vi "LB_AssertDisabledItems_Tests.vi"(11 "error in":errorcluster) -> (15 "error out":errorcluster)   [LabVIEW 2016, in "DronaTest.lvlib"]
uses:
  DronaTest.lvlib
  APIs/Stimulus/ControlValue/SetValueAuto.vi
  APIs/Assert/AssertControlValue/Controls/Listbox/AssertDisabledItems.vi
  <vilib>/addons/_JKI Toolkits/Caraya/classes/Assert/Assert Error.vi
  <vilib>/addons/_JKI Toolkits/Caraya/classes/Assert/Assert Equal Value_Variant.vi
  <vilib>/addons/_JKI Toolkits/Caraya/classes/Test/Test.lvclass
  Drona.lvlib
  <vilib>/SLL Toolkit/SLL Debug/SLL Debug.lvlib
  <vilib>/addons/_JKI Toolkits/Caraya/classes/Assert/Assert.lvclass
  APIs/Stimulus/ControlValue/ControlValue.lvlib
  APIs/Assert/AssertControlValue/Controls/Listbox/AssertListbox.lvlib
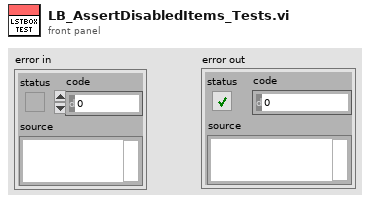
[diagram p1: front panel]
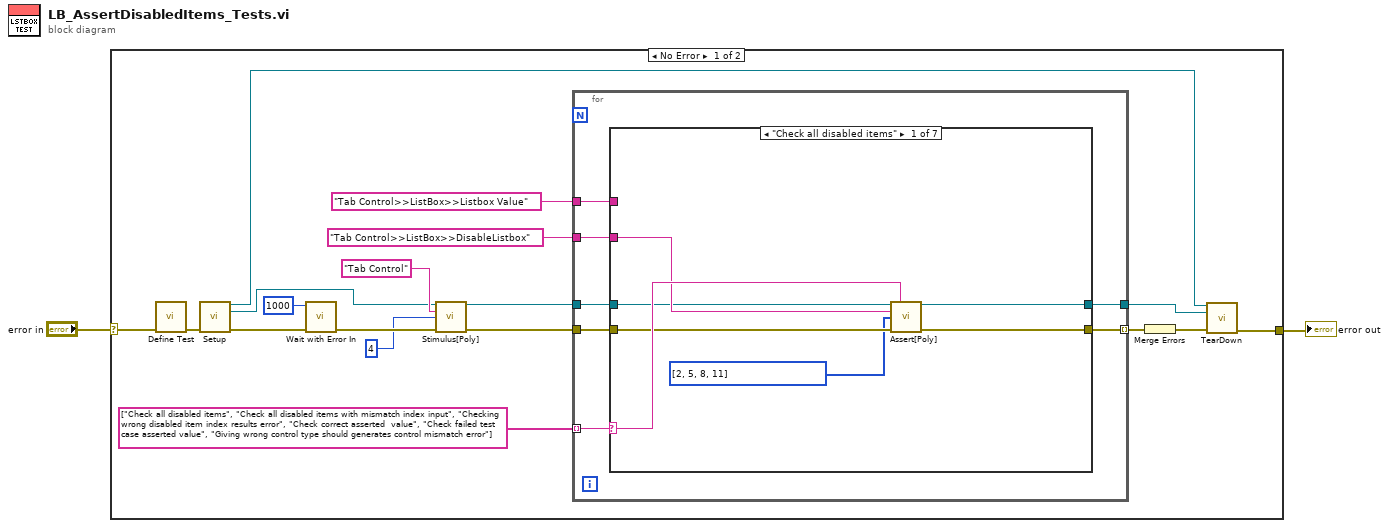
[diagram p0: block diagram]
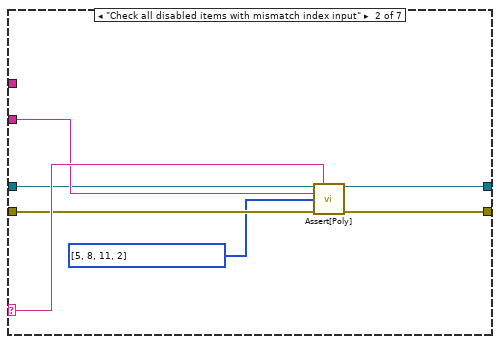
[diagram p2: hidden frame]
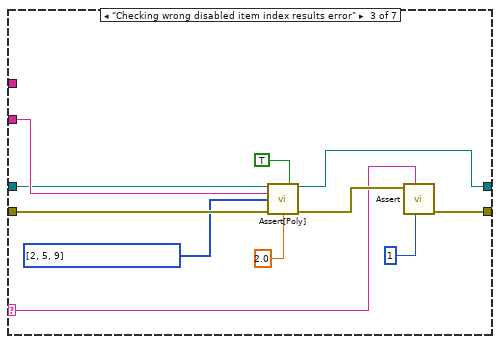
[diagram p3: hidden frame]
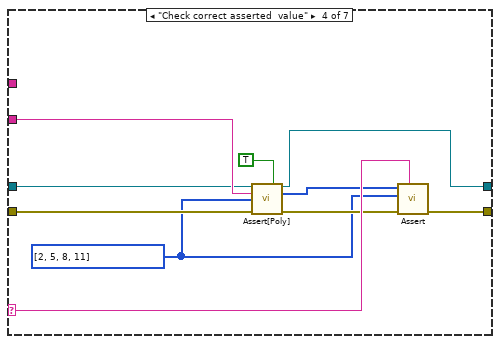
[diagram p4: hidden frame]
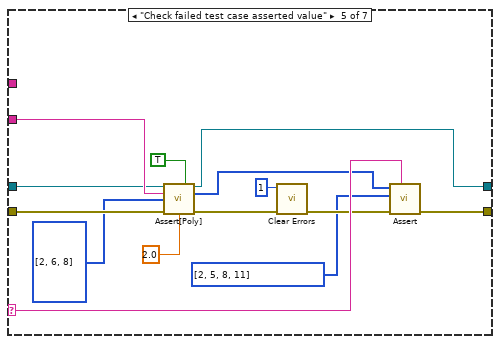
[diagram p5: hidden frame]
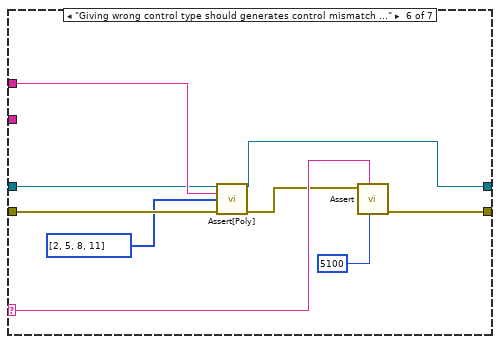
[diagram p6: hidden frame]
diagram:
  n1 = case shown="No Error" "error in" {
    selector: "error in" -> [w20 w88]
    tunnel: [w3 w88] -> w1
    frame No Error {
      n2 = call <vilib>:"Define Test.vi"("error in (no error)"=w20) -> ("error out"=w9:errorcluster)  [unwired: 9 in, 1 out]
      n3 = call "Setup.vi"("error in (no error)"=w9) -> ("Application Ref"=w5:refnum<vi>, "VI out"=w7:refnum<vi>, "error out"=w8:errorcluster)  [unwired: 12 in]
      n4 = call <vilib>:"Wait with Error In.vi"("error in (no error)"=w8, "milliseconds to wait"=u32 1000) -> ("error out"=w18:errorcluster)  [unwired: 9 in]
      n5 = call-poly "Stimulus[Poly].vi"("VI Reference In"=w7, "Control Path"="Tab Control", "Value (Signaling)"=4, "error in"=w18) -> ("VI Reference Out"=w14:refnum<vi>, "error out"=w17:errorcluster)  [unwired: 10 in]
      n6 = for {
        tunnel: w14 -> [w26]
        tunnel: "Tab Control>>ListBox>>DisableListbox" ("Control Path") -> [w25]
        tunnel: "Tab Control>>ListBox>>Listbox Value" ("Control Path") -> [w24]
        tunnel: string[] ["Check all disabled items", "Check all disabled items with mismatch index input", "Checking wrong disabled item index results error", "Check correct asserted  value", "Check failed test case asserted value", "Giving wrong control type should generates control mismatch error"] -> [w22] mode=indexing
        tunnel: [w21] -> w4
        tunnel: w17 -> [w27]
        tunnel: [w23] -> w10 mode=indexing
        n7 = case shown="\"Check all disabled items\"" w22 {
          selector: w22 -> [w32 w39 w45 w61 w75 w84 _]
          tunnel: w27 -> [w30 w37 w51 w57 w71 w79 w87]
          tunnel: w26 -> [w29 w36 w50 w56 w70 w78 w86]
          tunnel: w25 -> [w31 w38 w52 w60 w74 _ _]
          tunnel: w24 -> [_ _ _ _ _ w81 _]
          tunnel: [w34 w41 w47 w62 w76 w85 w87] -> w23
          tunnel: [w33 w40 w44 w59 w73 w80 w86] -> w21
          frame "Check all disabled items" {
            n8 = call-poly "Assert[Poly].vi"("VI Reference In"=w29, "Test Label"=w32, "Control Path"=w31, "Disabled Items"=i32[] [2, 5, 8, 11], "Error In"=w30) -> ("VI Reference Out"=w33:refnum<vi>, "Error Out"=w34:errorcluster)  [unwired: 8 in, 1 out]
          }
          frame "Check all disabled items with mismatch index input" {
            n9 = call-poly "Assert[Poly].vi"("VI Reference In"=w36, "Test Label"=w39, "Control Path"=w38, "Disabled Items"=i32[] [5, 8, 11, 2], "Error In"=w37) -> ("VI Reference Out"=w40:refnum<vi>, "Error Out"=w41:errorcluster)  [unwired: 8 in, 1 out]
          }
          frame "Checking wrong disabled item index results error" {
            n10 = call-poly "Assert[Poly].vi"("VI Reference In"=w50, "Assert Only? (F)"=TRUE, "Control Path"=w52, "Disabled Items"=i32[] [2, 5, 9], "Error In"=w51, "Timeout(5 sec)"=2.0) -> ("VI Reference Out"=w44:refnum<vi>, "Error Out"=w48:errorcluster)  [unwired: 7 in, 1 out]
            n11 = call-poly <vilib>:"Assert.vi"("error code (1)"=1, "Label"=w45, "Error?"=w48) -> ("error out"=w47:errorcluster)  [unwired: 7 in, 1 out]
          }
          frame "Check correct asserted  value" {
            w53 = i32[] [2, 5, 8, 11] ("Disabled Items")
            n12 = call-poly "Assert[Poly].vi"("VI Reference In"=w56, "Assert Only? (F)"=TRUE, "Control Path"=w60, "Disabled Items"=w53, "Error In"=w57) -> ("VI Reference Out"=w59:refnum<vi>, "Asserted Value"=w54:i32[], "Error Out"=w55:errorcluster)  [unwired: 8 in]
            n13 = call-poly <vilib>:"Assert.vi"("Label"=w61, "error in (no error)"=w55, "Y"=w53, "X"=w54) -> ("error out"=w62:errorcluster)  [unwired: 6 in, 1 out]
          }
          frame "Check failed test case asserted value" {
            n14 = call-poly "Assert[Poly].vi"("VI Reference In"=w70, "Assert Only? (F)"=TRUE, "Control Path"=w74, "Disabled Items"=i32[] [2, 6, 8], "Error In"=w71, "Timeout(5 sec)"=2.0) -> ("VI Reference Out"=w73:refnum<vi>, "Asserted Value"=w68:i32[], "Error Out"=w69:errorcluster)  [unwired: 7 in]
            n15 = call <vilib>:"Clear Errors.vi"("error in (no error)"=w69, "specific error code to clear (0: all)"=1) -> ("error out"=w67:errorcluster)  [unwired: 4 in, 1 out]
            n16 = call-poly <vilib>:"Assert.vi"("Label"=w75, "error in (no error)"=w67, "Y"=i32[] [2, 5, 8, 11] ("Disabled Items"), "X"=w68) -> ("error out"=w76:errorcluster)  [unwired: 6 in, 1 out]
          }
          frame "Giving wrong control type should generates control mismatch error" {
            n17 = call-poly "Assert[Poly].vi"("VI Reference In"=w78, "Control Path"=w81, "Disabled Items"=i32[] [2, 5, 8, 11], "Error In"=w79) -> ("VI Reference Out"=w80:refnum<vi>, "Error Out"=w82:errorcluster)  [unwired: 9 in, 1 out]
            n18 = call-poly <vilib>:"Assert.vi"("error code (1)"=5100, "Label"=w84, "Error?"=w82) -> ("error out"=w85:errorcluster)  [unwired: 7 in, 1 out]
          }
          frame Default {
          }
        }
      }
      n19 = Merge Errors(w10) -> (w6:errorcluster)
      n20 = call "TearDown.vi"("Application Ref"=w5, "VI in"=w4, "error in (no error)"=w6) -> ("error out"=w3:errorcluster)  [unwired: 12 in]
    }
    frame Error {
    }
  }
  "error out" <- w1
